vi "State Change.vi"(6 "Setup":bool, 8 "error in":errorcluster, 9 "Start":bool, 10 "Run Selector":bool, 11 "stop":bool) -> (0 "error IO":errorcluster, 5 "Next State":T1)   [LabVIEW 2013]
doc: "This sub VI is deciding the next state of the VI according to the boolean input of \nStop,Run Selector,Start and Setup."
uses:
  Controls/Sprinkler State.ctl
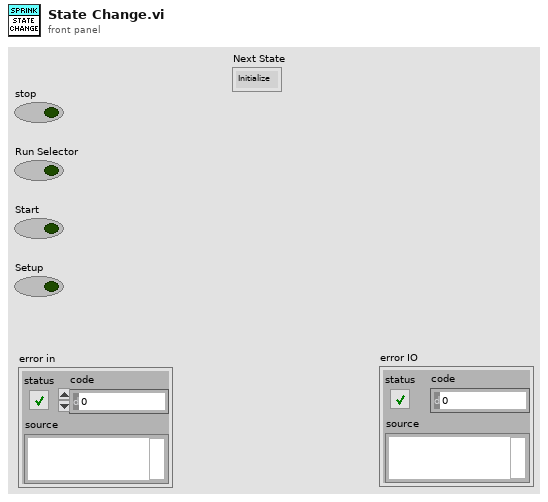
[diagram p1: front panel]
types:
  T1 = typedef "Sprinkler State.ctl" = enum16{"Initialize", "Setup", "Select", "Single", "Continous", "Start", "Stop"}
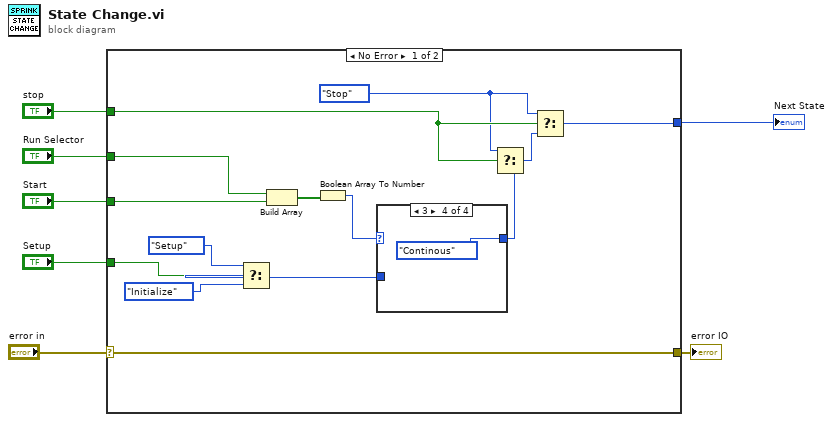
[diagram p0: block diagram]
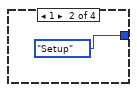
[diagram p3: hidden frame]
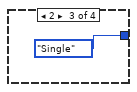
[diagram p4: hidden frame]
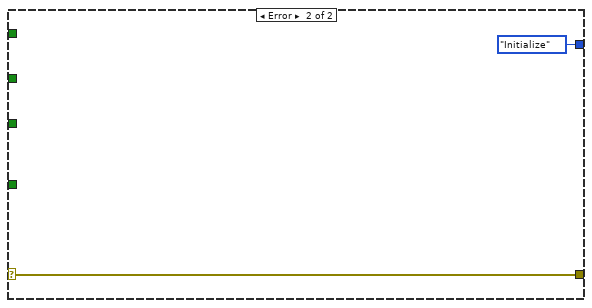
[diagram p5: hidden frame]
diagram:
  n1 = case shown="No Error" "error in" {
    selector: "error in" -> [w9 w27]
    tunnel: "Run Selector" -> [w17 _]
    tunnel: "Start" -> [w16 _]
    tunnel: "stop" -> [w14 _]
    tunnel: "Setup" -> [w11 _]
    tunnel: [w10 Sprinkler_State."Initialize" ("Next State")] -> w3
    tunnel: [w9 w27] -> w1
    frame No Error {
      w8 = Sprinkler_State."Stop"
      n2 = Select(t=Sprinkler_State."Setup" ("Next State"), s=w11, f=Sprinkler_State."Initialize" ("Next State")) -> (s? t:f=w20:T1)
      n3 = Build Array(w17, w16) -> (w18:bool[])
      n4 = Boolean Array To Number(Boolean array=w18) -> (number=w19:u32)
      n5 = case shown="3" w19 {
        tunnel: [w22 Sprinkler_State."Setup" ("Next State") Sprinkler_State."Single" ("Next State") Sprinkler_State."Continous" ("Next State")] -> w21
        tunnel: w20 -> [w22 _ _ _]
        frame 0, Default {
        }
        frame 1 {
        }
        frame 2 {
        }
        frame 3 {
        }
      }
      n6 = Select(t=w8, s=w14, f=w21) -> (s? t:f=w15:T1)
      n7 = Select(t=w8, s=w14, f=w15) -> (s? t:f=w10:T1)
    }
    frame Error {
    }
  }
  "Next State" <- w3
  "error IO" <- w1
